vi "Create VI Name - Dep array.vi"(8 "error in (no error)":errorcluster, 9 "Container - Regex pairs":T1=[{"Container to create"="TEST", "Regex"="^test_.*\\.vi"}, {"Container to create"="TEST", "Regex"="_test.vi$"}, {"Container to create"="DRV", "Regex"="^DRV_.*\\.lv.*$"}, {"Container to create"="HWT", "Regex"="^HWT_.*\\.lv.*$"}, {"Container to create"="FCN", "Regex"="^FCN_.*\\.lv.*$"}, {"Container to create"="INS", "Regex"="^INS_.*\\.lv.*$"}], 10 "Groupings":T2={"Group vi.lib"=FALSE, "Group instr.lib"=FALSE, "Group user.lib"=FALSE, "Group All LabVIEW"=FALSE, "Make Custom Containers"=TRUE, "Ignore LabVIEW directory"=FALSE}, 11 "All Files in Dir":path[](array[path])) -> (0 "error out":errorcluster, 2 "Name-Dep Array":T3[](array[typedef]))   [LabVIEW 2018, in "Shared Dependencies.lvlib"]
uses:
  Shared Dependencies.lvlib
  Name and Dependency processing/Name - Dep Cluster.ctl
  Grouping Control.ctl
  Container - Regex array.ctl
  Name and Dependency processing/Name and Dependency Processing.lvlib
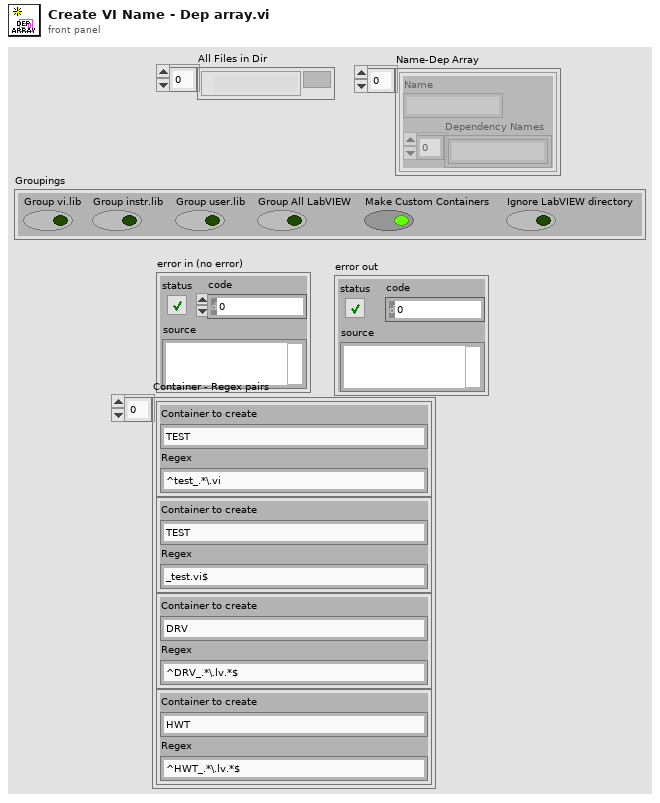
[diagram p1: front panel]
types:
  T1 = typedef "Shared Dependencies.lvlib/Container - Regex array.ctl" = cluster{"Container to create":string, "Regex":string}[]
  T2 = typedef "Name and Dependency Processing.lvlib/Grouping Control.ctl" = cluster{"Group vi.lib":bool, "Group instr.lib":bool, "Group user.lib":bool, "Group All LabVIEW":bool, "Make Custom Containers":bool, "Ignore LabVIEW directory":bool}
  T3 = typedef "Name and Dependency Processing.lvlib/Name - Dep Cluster.ctl" = cluster{"Name":string, "Dependency Names":string[]}
  T4 = typedef "Name and Dependency Processing.lvlib/Dep Names and Paths.ctl" = cluster{"Dependency Names":string[], "Dependency Paths":path[]}
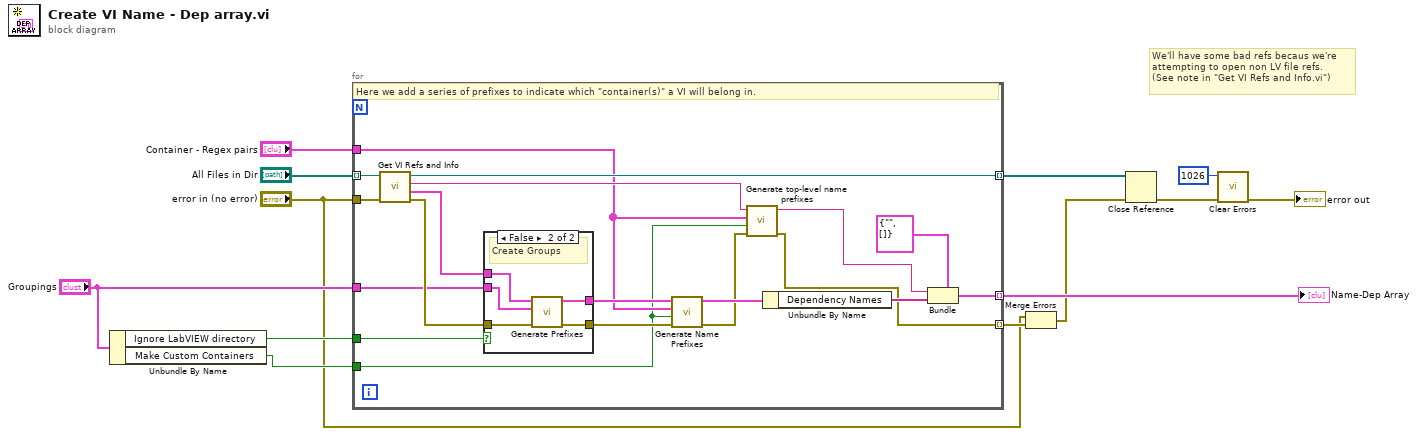
[diagram p0: block diagram]
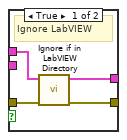
[diagram p2: hidden frame]
diagram:
  # "We'll have some bad refs becaus we're\nattempting to open non LV file refs.\n(See note in \"Get VI Refs and Info.vi\")"
  n1 = Unbundle By Name("Groupings") -> ("Ignore LabVIEW directory"=w3:bool, "Make Custom Containers"=w2:bool)
  n2 = for {
    tunnel: "All Files in Dir" -> [w32] mode=indexing
    tunnel: [w31] -> w13 mode=indexing
    tunnel: [w30] -> w11 mode=indexing
    tunnel: "error in (no error)" -> [w26]
    tunnel: w3 -> [w25]
    tunnel: "Groupings" -> [w24]
    tunnel: [w16] -> w10 mode=indexing
    tunnel: "Container - Regex pairs" -> [w15]
    tunnel: w2 -> [w14]
    # "Here we add a series of prefixes to indicate which \"container(s)\" a VI will belong in."
    n3 = call "Get VI Refs and Info.vi"("error in (no error)"=w26, "Path to analyze"=w32) -> ("error out"=w28:errorcluster, "output cluster"=w29:T4, "Name"=w19:string, "VI out"=w30:refnum<vi>)  [unwired: 6 in]
    n4 = case shown="False" w25 {
      tunnel: [w36 w38] -> w21
      tunnel: w29 -> [w35 w40]
      tunnel: w28 -> [w34 w37]
      tunnel: [w33 w41] -> w22
      tunnel: w24 -> [_ w39]
      frame True {
        # "Ignore LabVIEW"
        n5 = call "Ignore if in LabVIEW Directory.vi"("error in"=w34, "Dep Names and Paths"=w35) -> ("error out"=w33:errorcluster, "Filtered Dep Names and Paths"=w36:T4)  [unwired: 8 in]
      }
      frame False {
        # "Create Groups"
        n6 = call "Generate Prefixes.vi"("error in (no error)"=w37, "Groupings"=w39, "Dep Names and Paths"=w40) -> ("error out"=w41:errorcluster, "Prefixed Dep Names and Paths"=w38:T4)  [unwired: 7 in]
      }
    }
    n7 = call "Generate Name Prefixes.vi"("error in"=w22, "Add Prefix?"=w14, "Container - Regex pairs"=w15, "Dep Names and Paths"=w21) -> ("error out"=w17:errorcluster, "Prefixed Dep Names and Paths"=w20:T4)  [unwired: 6 in]
    n8 = call "Generate top-level name prefixes.vi"("error in"=w17, "Add Prefix?"=w14, "Container - Regex pairs"=w15, "String"=w19) -> ("error out"=w16:errorcluster, "element"=w18:string)  [unwired: 6 in]
    n9 = Unbundle By Name(w20) -> ("Dependency Names"=w27:string[])
    n10 = Bundle(cluster=T3 {"Name"="", "Dependency Names"=[]}, "Name"=w18, "Dependency Names"=w27) -> (w31:T3)
  }
  "Name-Dep Array" <- w13
  n11 = Merge Errors("error in (no error)", w10) -> (w9:errorcluster)
  n12 = Close Reference(reference=w11, error in (no error)=w9) -> (error out=w7:errorcluster)
  n13 = call <vilib>:"Clear Errors.vi"("error in (no error)"=w7, "specific error code to clear (0: all)"=1026) -> ("error out"=→"error out":errorcluster)  [unwired: 4 in, 1 out]
